vi "ROI_test.vi"() -> ()   [LabVIEW 2015]
doc: "This VI is used to test the ROI selection function."
uses:
  <vilib>/Utility/miscctls.llb/LVPoint32TypeDef.ctl
  <vilib>/Utility/miscctls.llb/LVPositionTypeDef.ctl
  inputImages.ctl
panel:
  out "Position":T1
  out "MouseUp":T2
  in  "Stop":bool
  out "MouseDown":T2
  out "Image":picture
  in  "Width":i32=1280
  in  "ColumnStart":i32=1000
  in  "Height":i32=1024
  in  "RowStart":i32=800
  in  "Input_Z":dbl[](array[numeric])=[1.0, 2.0, 3.0, 4.0]
  out "Elapsed time (s)":dbl
  in  "Image4":path=path "C:/Users/Administrator/Desktop/focus/3.png"
  in  "Image3":path=path "C:/Users/Administrator/Desktop/focus/2.png"
  in  "Image2":path=path "C:/Users/Administrator/Desktop/focus/1.png"
  out "BestPosition":dbl
  in  "Image1":path=path "C:/Users/Administrator/Desktop/focus/0.png"
  # "This VI is used to test the ROI \nselection function."
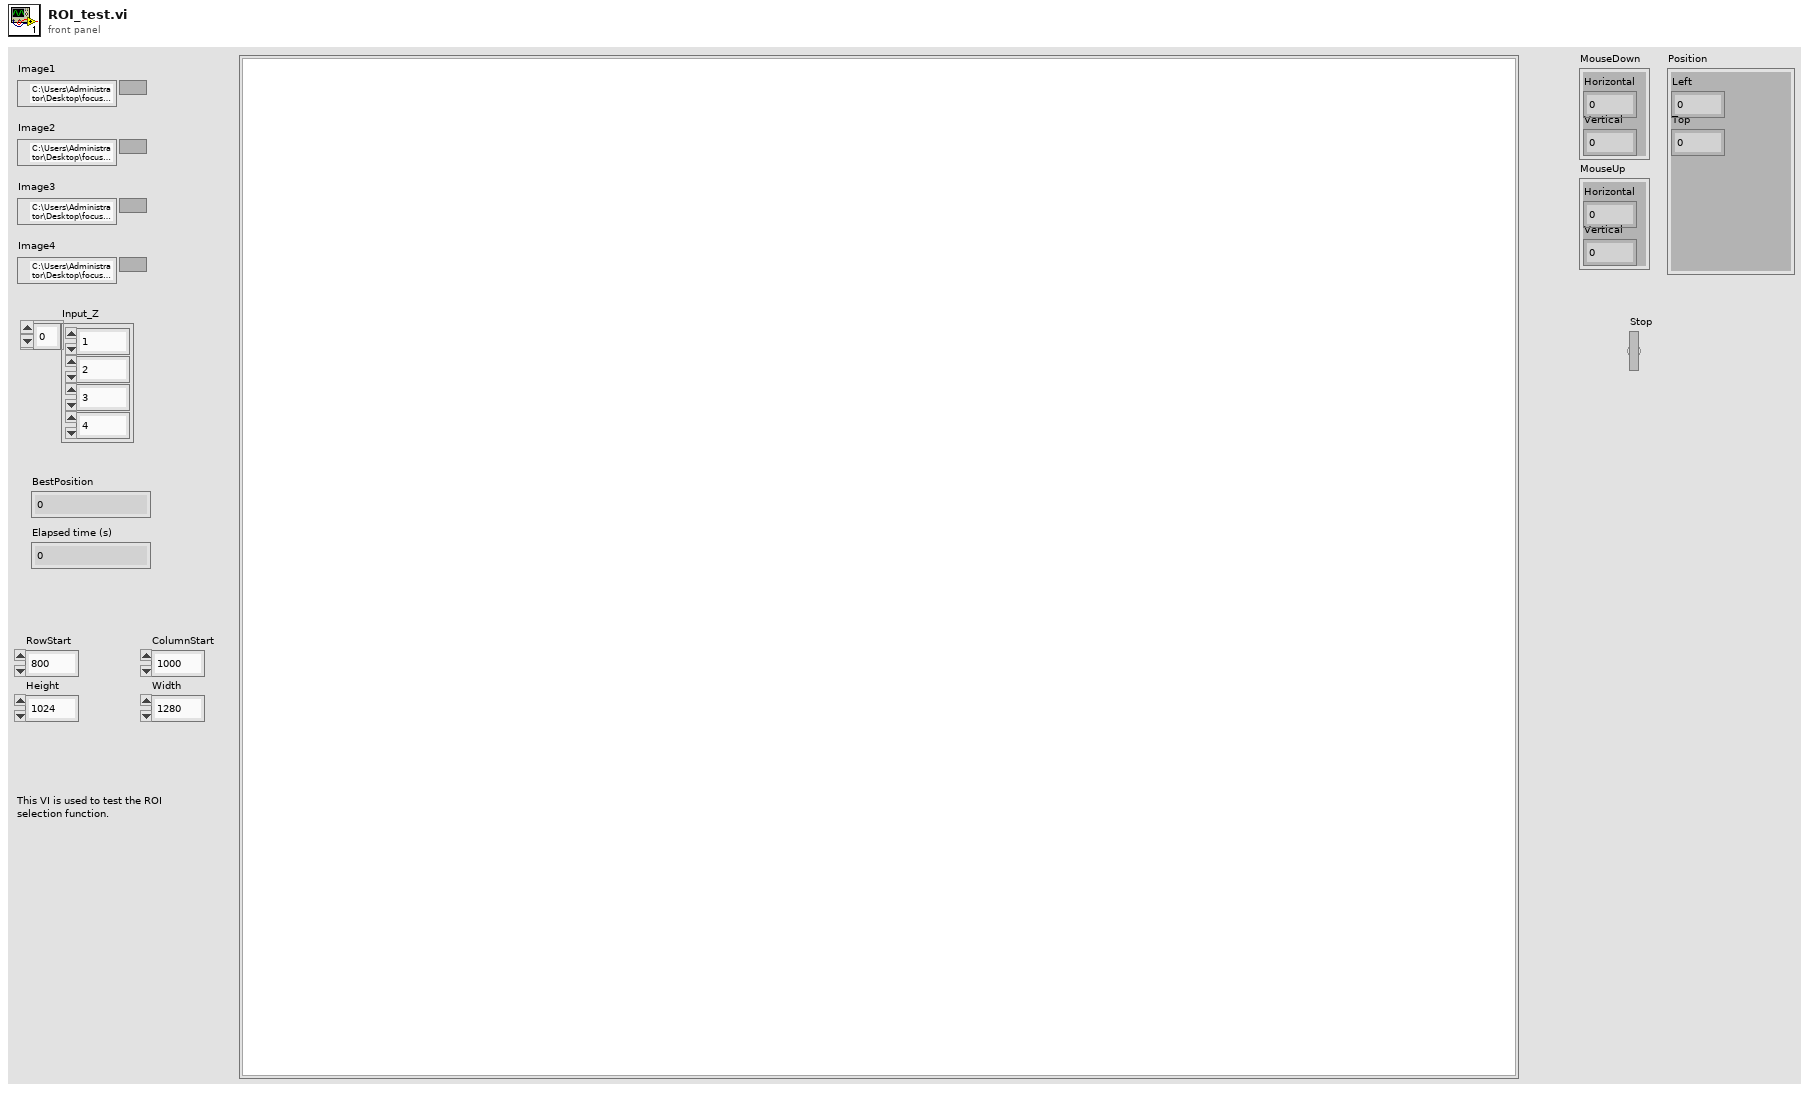
[diagram p1: front panel]
types:
  T1 = typedef "LVPositionTypeDef.ctl" = cluster{"Left":i32, "Top":i32}
  T2 = typedef "LVPoint32TypeDef.ctl" = cluster{"Horizontal":i32, "Vertical":i32}
  T3 = typedef "imagedata.ctl" = cluster{"image type":i32, "image depth":i32, "image":u8[], "mask":u8[], "colors":u32[], "Rectangle":cluster{"left":i16, "top":i16, "right":i16, "bottom":i16}}
  T4 = typedef "inputImages.ctl" = cluster{"Image2":u8[][], "Image3":u8[][], "Image4":u8[][], "Image1":u8[][]}
  T5 = cluster{"left":i16, "top":i16, "right":i16, "bottom":i16}
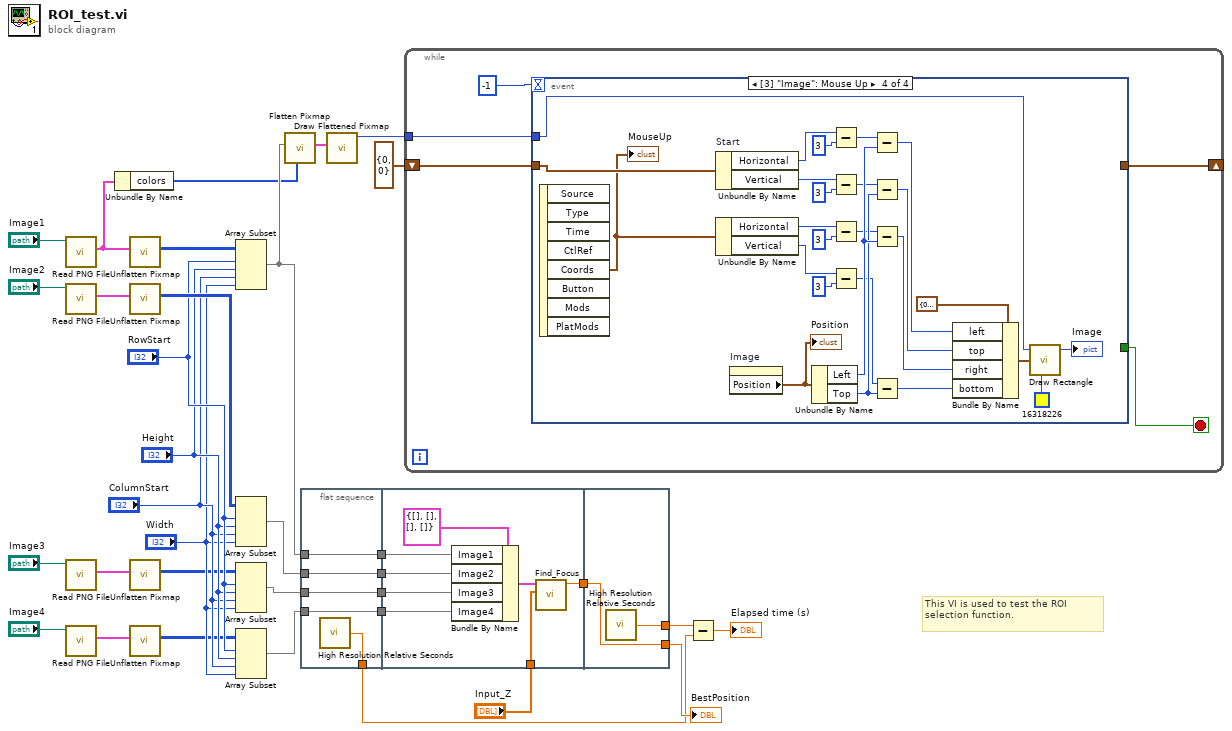
[diagram p0: block diagram]
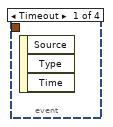
[diagram p2: hidden frame]
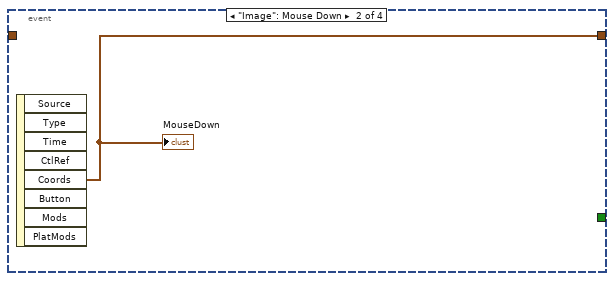
[diagram p3: hidden frame]
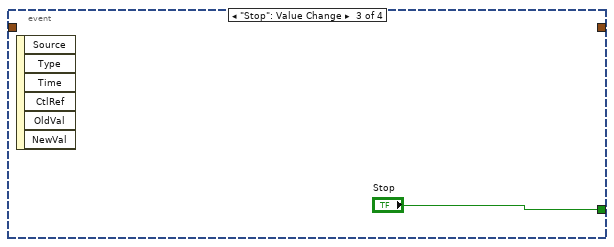
[diagram p4: hidden frame]
diagram:
  # "This VI is used to test the ROI \nselection function."
  n1 = call <vilib>:"Read PNG File.vi"("path to PNG file"="Image1") -> ("image data"=w4:T3)  [unwired: 8 in, 2 out]
  n2 = call <vilib>:"Read PNG File.vi"("path to PNG file"="Image2") -> ("image data"=w33:T3)  [unwired: 8 in, 2 out]
  n3 = call <vilib>:"Read PNG File.vi"("path to PNG file"="Image3") -> ("image data"=w30:T3)  [unwired: 8 in, 2 out]
  n4 = call <vilib>:"Read PNG File.vi"("path to PNG file"="Image4") -> ("image data"=w29:T3)  [unwired: 8 in, 2 out]
  n5 = Unbundle By Name(w4) -> ("colors"=w3:u32[])
  n6 = call <vilib>:"Unflatten Pixmap.vi"("image data"=w4) -> ("8-bit pixmap"=w7:u8[][])  [unwired: 4 in, 6 out]
  n7 = call <vilib>:"Unflatten Pixmap.vi"("image data"=w33) -> ("8-bit pixmap"=w17:u8[][])  [unwired: 4 in, 6 out]
  n8 = call <vilib>:"Unflatten Pixmap.vi"("image data"=w30) -> ("8-bit pixmap"=w11:u8[][])  [unwired: 4 in, 6 out]
  n9 = call <vilib>:"Unflatten Pixmap.vi"("image data"=w29) -> ("8-bit pixmap"=w9:u8[][])  [unwired: 4 in, 6 out]
  n10 = Array Subset(array=w7, index (row)="RowStart", length (row)="Height", index (col)="ColumnStart", length (col)="Width") -> (w5:u8[][])
  n11 = Array Subset(array=w17, index (row)="RowStart", length (row)="Height", index (col)="ColumnStart", length (col)="Width") -> (w16:u8[][])
  n12 = Array Subset(array=w11, index (row)="RowStart", length (row)="Height", index (col)="ColumnStart", length (col)="Width") -> (w10:u8[][])
  n13 = Array Subset(array=w9, index (row)="RowStart", length (row)="Height", index (col)="ColumnStart", length (col)="Width") -> (w8:u8[][])
  n14 = call <vilib>:"Flatten Pixmap.vi"("colors"=w3, "8-bit pixmap"=w5) -> ("image data"=w6:T3)  [unwired: 9 in]
  n15 = flat-sequence {
    tunnel: w8 -> [w36]
    tunnel: w10 -> [w37]
    tunnel: w16 -> [w38]
    tunnel: w5 -> [w39]
    tunnel: [w39] -> w25
    tunnel: [w38] -> w24
    tunnel: [w37] -> w23
    tunnel: [w36] -> w22
    tunnel: [w35] -> w19
    tunnel: [w47] -> w26
    tunnel: w25 -> [w45]
    tunnel: w24 -> [w44]
    tunnel: w23 -> [w43]
    tunnel: w22 -> [w42]
    tunnel: "Input_Z" -> [w40]
    tunnel: [w49] -> w27
    tunnel: w26 -> [w49]
    tunnel: [w48] -> w20
    frame #0 {
      n16 = call <vilib>:"High Resolution Relative Seconds.vi"() -> ("relative seconds"=w35:dbl)
    }
    frame #1 {
      n17 = Bundle By Name(cluster=T4 {"Image2"=[], "Image3"=[], "Image4"=[], "Image1"=[]} ("Imput images"), "Image1"=w45, "Image2"=w44, "Image3"=w43, "Image4"=w42) -> (w41:T4)
      n18 = call "Find_Focus.vi"("Input_Z"=w40, "Imput images"=w41) -> ("BestPosition"=w47:dbl)  [unwired: 8 in, 1 out]
    }
    frame #2 {
      n19 = call <vilib>:"High Resolution Relative Seconds.vi"() -> ("relative seconds"=w48:dbl)
    }
  }
  n20 = call <vilib>:"Draw Flattened Pixmap.vi"("image data"=w6) -> ("new picture"=w1:picture)  [unwired: 8 in]
  n21 = while {
    shift-right: [w52] -> _
    shift-left: T2 {"Horizontal"=0, "Vertical"=0} ("Coords") -> [w51]
    tunnel: w1 -> [w50]
    stop <- w53 stop-if-true
    n22 = event shown="[3] \"Image\": Mouse Up" {
      selector: _ -> [_ _ _ _]
      dyn-events: _ -> [_ _ _ _]
      timeout: -1 -> [_ _ _ _]
      tunnel: [_ _ "Stop" _] -> w53
      tunnel: [_ w55 _ _] -> w52
      tunnel: w51 -> [_ _ _ w82]
      tunnel: w50 -> [_ _ _ w78]
      event Timeout {
        n23 = event-data() -> ()  [unwired: 1 in, 3 out]
      }
      event "Image": Mouse Down {
        n24 = event-data() -> ("Coords"=w55:T2)  [unwired: 1 in, 7 out]
        "MouseDown" <- w55
      }
      event "Stop": Value Change {
        n25 = event-data() -> ()  [unwired: 1 in, 6 out]
      }
      event "Image": Mouse Up {
        n26 = event-data() -> ("Coords"=w81:T2)  [unwired: 1 in, 7 out]
        "MouseUp" <- w81
        n27 = Unbundle By Name "Start"(w82) -> ("Horizontal"=w69:i32, "Vertical"=w66:i32)
        n28 = Unbundle By Name(w81) -> ("Horizontal"=w63:i32, "Vertical"=w60:i32)
        n29 = property on="Image" class="Pict"() -> ("Position"=w70:T1)  [unwired: 2 in, 2 out]
        "Position" <- w70
        n30 = Unbundle By Name(w70) -> ("Left"=w75:i32, "Top"=w72:i32)
        n31 = Subtract(x=w69, y=3) -> (x-y=w67:i32)
        n32 = Subtract(x=w66, y=3) -> (x-y=w65:i32)
        n33 = Subtract(x=w63, y=3) -> (x-y=w61:i32)
        n34 = Subtract(x=w60, y=3) -> (x-y=w58:i32)
        n35 = Subtract(x=w67, y=w75) -> (x-y=w76:i32)
        n36 = Subtract(x=w65, y=w72) -> (x-y=w73:i32)
        n37 = Subtract(x=w61, y=w75) -> (x-y=w74:i32)
        n38 = Subtract(x=w58, y=w72) -> (x-y=w71:i32)
        n39 = Bundle By Name(cluster=T5 {"left"=0, "top"=0, "right"=0, "bottom"=0} ("rect"), "left"=w76, "top"=w73, "right"=w74, "bottom"=w71) -> (w79:T5)
        n40 = call <vilib>:"Draw Rectangle.vi"("picture"=w78, "rect"=w79, "color(black)"=u32 16318226) -> ("new picture"=→"Image":picture)  [unwired: 6 in]
      }
    }
  }
  n41 = Subtract(x=w20, y=w19) -> (x-y=→"Elapsed time (s)":dbl)
  "BestPosition" <- w27
